vi "Create duplicate image buffer.vi"(8 "error in (no error)":errorcluster, 10 "String":string, 11 "Refnum in":T1) -> (0 "error out":errorcluster, 3 "Refnum out":T1)   [LabVIEW 2020]
uses:
  <vilib>/vision/Image Controls.llb/IMAQ Image.ctl
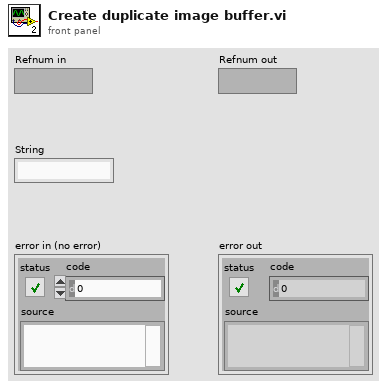
[diagram p1: front panel]
types:
  T1 = typedef "IMAQ Image.ctl" = refnum<image>
  T2 = typedef "Image Type" = u32
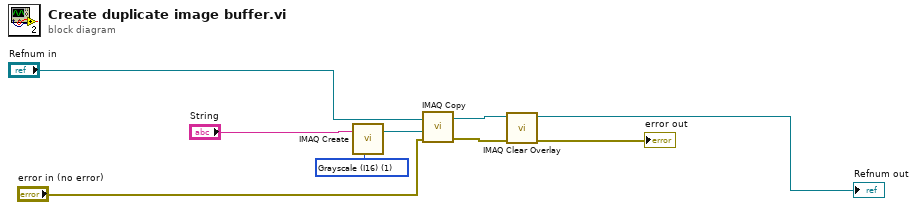
[diagram p0: block diagram]
diagram:
  w1 = T2 1 items=["Grayscale (U8)", "Grayscale (I16)", "Grayscale (SGL)", "Complex (CSG)", "RGB (U32)", "HSL (U32)", "RGB (U64)", "Grayscale (U16)"] ("Image Type")
  n1 = call "IMAQ Create"("Image Name"="String", "Image Type"=w1) -> ("New Image"=w2:T1)  [unwired: 3 in, 1 out]
  n2 = call "IMAQ Copy"("error in (no error)"="error in (no error)", "Image Dst"=w2, "Image Src"="Refnum in") -> ("error out"=w9:errorcluster, "Image Dst Out"=w5:T1)  [unwired: 3 in]
  n3 = call "IMAQ Clear Overlay"("error in (no error)"=w9, "Image"=w5) -> ("error out"=→"error out":errorcluster, "Image Out"=→"Refnum out":T1)  [unwired: 8 in]
